vi "Type Conversion.vi"() -> ()   [LabVIEW 2019]
panel:
  out "Indicator 4":string
  out "Indicator 3":bool
  out "Indicator 2":i32
  out "Indicator 1":dbl
  in  "Control 4":string="hello"
  in  "Control 3":bool
  in  "Control 2":i32=42
  in  "Control 1":dbl=3.0
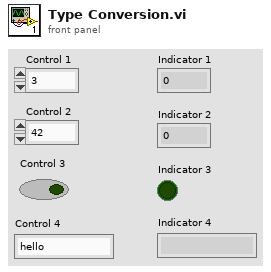
[diagram p1: front panel]
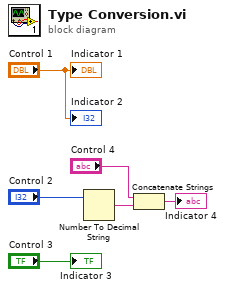
[diagram p0: block diagram]
diagram:
  n1 = Number To Decimal String(number="Control 2") -> (decimal integer string=w1:string)  [unwired: 1 in]
  n2 = Concatenate Strings("Control 4", w1) -> (→"Indicator 4":string)
  "Indicator 1" <- "Control 1"
  "Indicator 2" <- "Control 1"
  "Indicator 3" <- "Control 3"
